vi "Get 2dStringArray.vi"(8 "error in (no error)":errorcluster, 11 "2dStringArrayMsg In":refnum<class "2dStringArrayMsg.lvclass">) -> (0 "error out":errorcluster, 2 "Message Data":string[][](array[string]), 3 "2dStringArrayMsg Out":refnum<class "2dStringArrayMsg.lvclass">)   [LabVIEW 2009, in "LapDog.Messaging.v2.NativeArrays.lvlib" / "2dStringArrayMsg.lvclass"]
doc: "Returns the data contained in the message.\n\nThis method executes regardless of the error in state."
uses:
  2dStringArrayMsg.lvclass
  2dStringArrayMsg.lvclass/2dStringArrayMsg.ctl
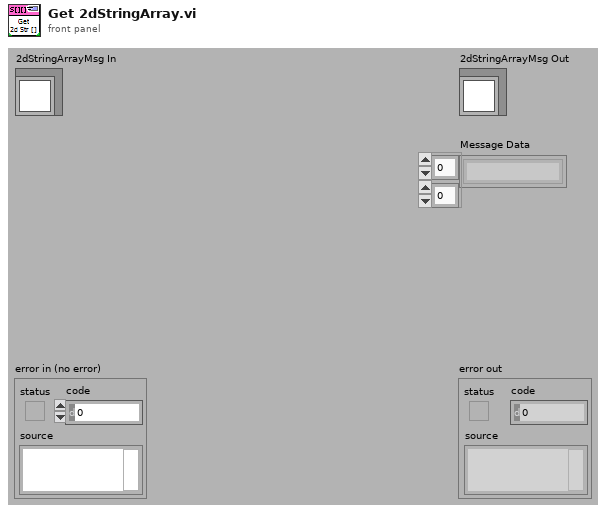
[diagram p1: front panel]
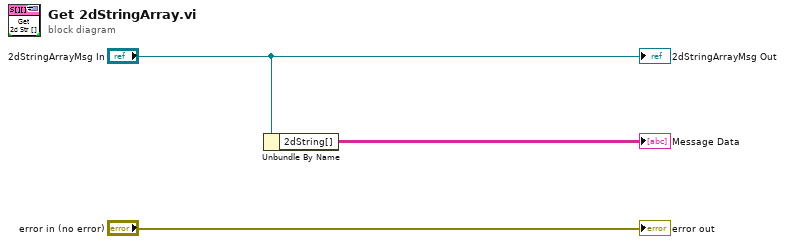
[diagram p0: block diagram]
diagram:
  n1 = Unbundle By Name("2dStringArrayMsg In") -> ("2dString[]"=→"Message Data":string[][])
  "error out" <- "error in (no error)"
  "2dStringArrayMsg Out" <- "2dStringArrayMsg In"
